vi "Read StateSim.vi"(8 "error in (no error)":errorcluster, 11 "MotorSim in":refnum<class "MotorSim.lvclass">) -> (0 "error out":errorcluster, 2 "StateSim":refnum<class "StateManager.lvclass">, 3 "MotorSim out":refnum<class "MotorSim.lvclass">, 5 "simEnum":T1(ring))   [LabVIEW 2018, in "MotorSim.lvclass"]
uses:
  MotorSim.lvclass
  StateManager/StateManager.lvclass
  MotorSim.lvclass/MotorSim.ctl
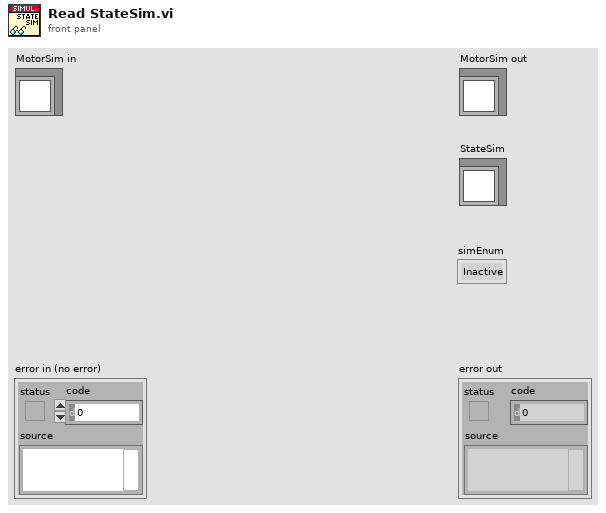
[diagram p1: front panel]
types:
  T1 = enum16{"Inactive", "IdleSim", "ReadySim", "WaitCCWlim", "WaitCWlim", "Homing", "Moving", "Stopping", "WaitValid", "WaitStop"}
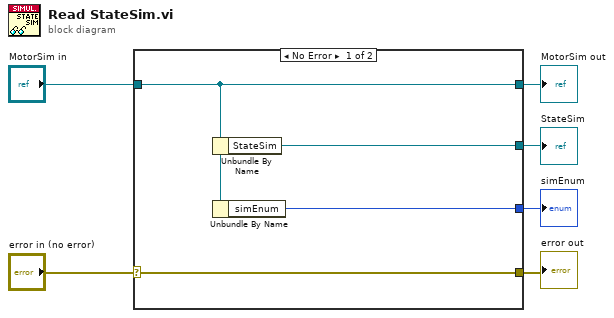
[diagram p0: block diagram]
diagram:
  n1 = case shown="No Error" "error in (no error)" {
    selector: "error in (no error)" -> [w10 w11]
    tunnel: [w10 w11] -> w5
    tunnel: [w8 w12] -> w3
    tunnel: "MotorSim in" -> [w8 w12]
    tunnel: [w9 _] -> w2
    tunnel: [w7 _] -> w1
    frame No Error {
      n2 = Unbundle By Name(w8) -> ("StateSim"=w9:refnum<class "StateManager.lvclass">)
      n3 = Unbundle By Name(w8) -> ("simEnum"=w7:T1)
    }
    frame Error {
    }
  }
  "error out" <- w5
  "MotorSim out" <- w3
  "StateSim" <- w2
  "simEnum" <- w1
